vi "Gaussian surface with offset model2.vi"(3 "output control":T1, 4 "data":variant, 5 "X":dbl[](array[numeric]), 6 "a":dbl[](array[numeric])) -> (0 "error out":errorcluster, 1 "f'(X,a)":dbl[][](array[numeric]), 2 "f(X,a)":dbl[](array[numeric]))   [LabVIEW 2015]
doc: "Gaussian surface with offset model"
uses:
  <vilib>/gmath/NumericalOptimization/LM_output select.ctl
  <vilib>/gmath/NI_Gmath.lvlib
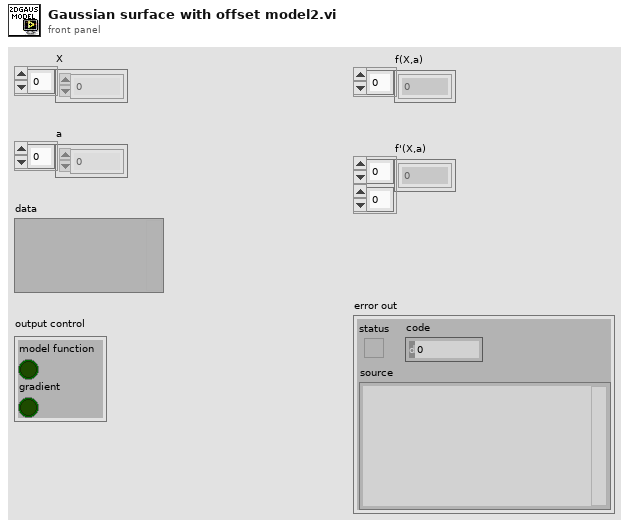
[diagram p1: front panel]
types:
  T1 = typedef "NI_Gmath.lvlib/LM_output select.ctl" = cluster{"model function":bool, "gradient":bool}
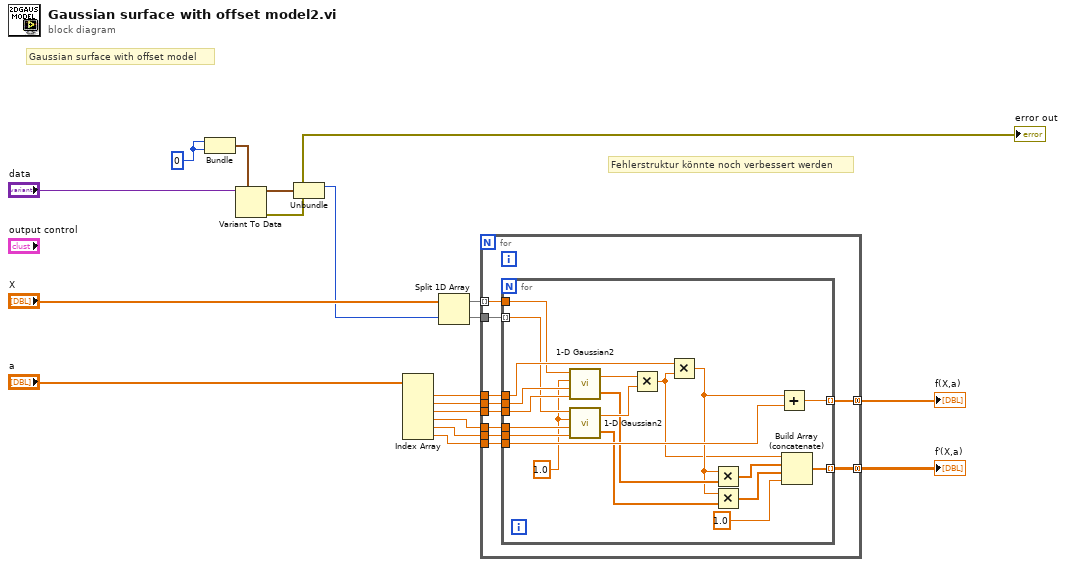
[diagram p0: block diagram]
diagram:
  w13 = 0
  # "Fehlerstruktur könnte noch verbessert werden"
  # "Gaussian surface with offset model"
  n1 = Bundle(w13, w13) -> (w7:cluster{i32, i32})  [unwired: 1 out]
  n2 = Variant To Data(type=w7, Variant="data") -> (data=w3:cluster{i32, i32}, error out=→"error out":errorcluster)  [unwired: 1 in]
  n3 = Unbundle(w3) -> (w2:i32)  [unwired: 1 out]
  n4 = Index Array(array="a") -> (element #1=w18:dbl, element #2=w17:dbl, element #3=w16:dbl, element #4=w10:dbl, element #5=w9:dbl, element #6=w8:dbl)  [unwired: 6 in]
  n5 = Split 1D Array(array="X", index=w2) -> (first subarray=w12:dbl[], second subarray=w11:dbl[])
  n6 = for {
    tunnel: w18 -> [w28]
    tunnel: w17 -> [w27]
    tunnel: w16 -> [w26]
    tunnel: w10 -> [w23]
    tunnel: w9 -> [w22]
    tunnel: w8 -> [w21]
    tunnel: w12 -> [w25] mode=indexing
    tunnel: w11 -> [w24]
    tunnel: [w20] -> w5 mode=concatenating
    tunnel: [w19] -> w4 mode=concatenating
    n7 = for {
      tunnel: [w47] -> w20 mode=indexing
      tunnel: w28 -> [w48]
      tunnel: w27 -> [w46]
      tunnel: w26 -> [w45]
      tunnel: w25 -> [w44]
      tunnel: w24 -> [w43] mode=indexing
      tunnel: w23 -> [w42]
      tunnel: w22 -> [w41]
      tunnel: w21 -> [w40]
      tunnel: [w36] -> w19 mode=indexing
      w39 = 1.0 ("a")
      n8 = call "1-D Gaussian2.vi"("sigma"=w45, "m"=w46, "a"=w39, "x"=w44) -> ("y'"=w35:dbl[], "y"=w38:dbl)
      n9 = call "1-D Gaussian2.vi"("sigma"=w41, "m"=w42, "a"=w39, "x"=w43) -> ("y'"=w33:dbl[], "y"=w37:dbl)
      n10 = Multiply(x=w38, y=w37) -> (x*y=w29:dbl)
      n11 = Multiply(x=w48, y=w29) -> (x*y=w30:dbl)
      n12 = Multiply(x=w30, y=w35) -> (x*y=w34:dbl[])
      n13 = Multiply(x=w30, y=w33) -> (x*y=w32:dbl[])
      n14 = Add(x=w30, y=w40) -> (x+y=w47:dbl)
      n15 = Build Array (concatenate)(w29, w34, w32, 1.0) -> (w36:dbl[])
    }
  }
  "f(X,a)" <- w5
  "f'(X,a)" <- w4
